vi "CreateNew_Init.vi"(11 "Wizard":T1) -> (1 "Label":string, 2 "Enable Finish":bool, 3 "Enable Next":bool)   [LabVIEW 2020, in "FlexWorker_Provider.lvlib"]
uses:
  FlexWorker_Provider.lvlib
  <resource>/Framework/Providers/API/ItemRef.ctl
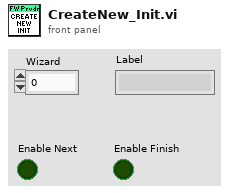
[diagram p1: front panel]
types:
  T1 = typedef "ItemRef.ctl" = u64
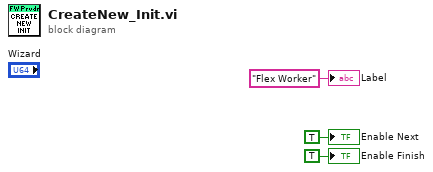
[diagram p0: block diagram]
diagram:
  "Enable Next" <- TRUE ("Enable Next")
  "Enable Finish" <- TRUE ("Enable Finish")
  "Label" <- "Flex Worker" ("Label")
